vi "File Compatibility Test.vi"() -> (0 "error out":errorcluster, 3 "result":string)   [LabVIEW 2014]
doc: "This test will find some issues caused by a modification to To and From string methods that don't support older configuration versions. The test finds and attempts to open all .pcfg files that it can find in the repo and returns details in a 'result' string if any of them fail."
uses:
  <vilib>/NI/Configuration Framework/class discovery singleton/class discovery singleton methods.ctl
  <vilib>/NI/DCAF/Tag Editor Core/Configuration Editor/Classes/SystemConfigRepo/SystemConfigRepo.lvclass
  <vilib>/NI/DCAF/Tag Editor Core/Framework Configuration Classes/class cache/PL_class cache.lvlib
  <vilib>/NI/Configuration Framework/class discovery singleton/class discovery singleton.lvlib
panel:
  out "All Files in Dir":path[](array[path])
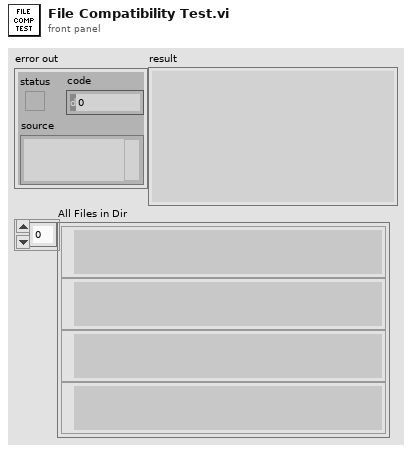
[diagram p1: front panel]
types:
  T1 = typedef "class discovery singleton.lvlib/class discovery singleton methods.ctl" = enum16{"add search paths", "load class by name", "list available classes", "get class path", "delete cache"}
  T2 = typedef "PL_class cache.lvlib/cache definition.ctl" = cluster{"configuration":T3, "class cache data":T4}
  T3 = typedef "PL_class cache.lvlib/cache search configuration.ctl" = cluster{"Search Paths":path[], "Folders to Exclude":string[], "full class list":path[]}
  T4 = typedef "PL_class cache.lvlib/cached class information.ctl" = cluster{"targets":T5[], "engines":T6[], "modules":T6[], "ignored class list":path[]}
  T5 = typedef "PL_class cache.lvlib/target class metadata.ctl" = cluster{"file name":string, "fully qualified name":string, "menu display name":string, "configuration class name":string}
  T6 = typedef "PL_class cache.lvlib/class metadata.ctl" = cluster{"file name":string, "fully qualified name":string, "menu display name":string, "configuration class":string, "category":string, "instances allowed":i32, "supported targets":T7[]}
  T7 = typedef "TBM configuration.lvclass/Target Types.ctl" = enum16{"Windows", "Mac", "Linux", "Linux RT ARM", "VxWorks", "Pharlap", "Other", "Linux RT x64"}
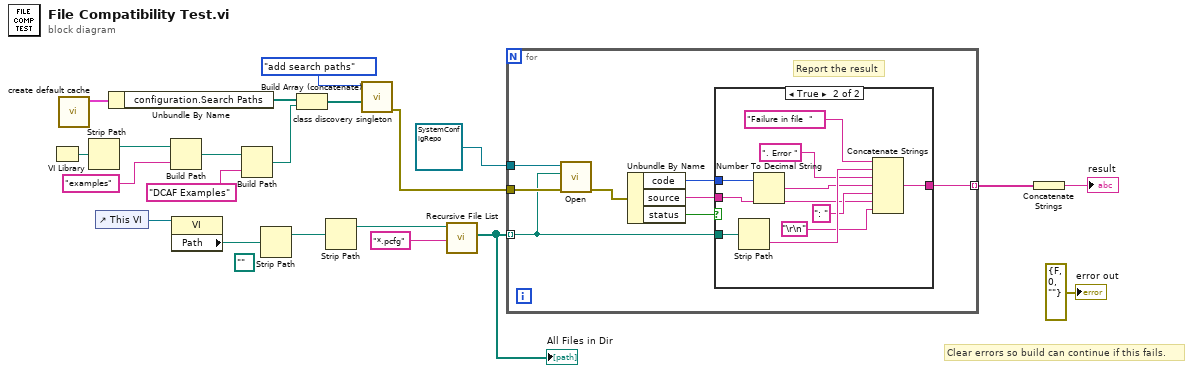
[diagram p0: block diagram]
diagram:
  (unwired) path "" ("VI Path")
  # "Clear errors so build can continue if this fails."
  n1 = VI Library() -> (path=w9:path)
  n2 = call <vilib>:"create default cache.vi"() -> ("cache"=w21:T2)  [unwired: 11 in]
  n3 = Strip Path(path=w9) -> (stripped path=w8:path)  [unwired: 1 out]
  n4 = control-ref of="This VI"() -> (w20:refnum<vi>)
  n5 = Unbundle By Name(w21) -> ("configuration.Search Paths"=w10:path[])
  n6 = Build Path(base path=w8, name or relative path="examples") -> (appended path=w6:path)
  n7 = property class="VI"(reference=w20) -> ("Path"=w19:path)  [unwired: 1 in, 2 out]
  n8 = Build Path(base path=w6, name or relative path="DCAF Examples") -> (appended path=w1:path)
  n9 = Strip Path(path=w19) -> (stripped path=w18:path)  [unwired: 1 out]
  n10 = Build Array (concatenate)(w10, w1) -> (w2:path[])
  n11 = Strip Path(path=w18) -> (stripped path=w17:path)  [unwired: 1 out]
  n12 = call <vilib>:"class discovery singleton.vi"("Plugin Search Paths"=w2, "method"=class_discovery_singleton_methods."add search paths") -> ("error out"=w3:errorcluster)  [unwired: 6 in, 3 out]
  n13 = call <vilib>:"Recursive File List.vi"("pattern"="*.pcfg", "Folder Path"=w17) -> ("All Files in Dir"=w15:path[])  [unwired: 5 in, 4 out]
  "All Files in Dir" <- w15
  n14 = for {
    tunnel: w3 -> [w29]
    tunnel: refnum<class "SystemConfigRepo.lvclass"> refnum ("repository out") -> [w28]
    tunnel: [w23] -> w13 mode=indexing
    tunnel: w15 -> [w22] mode=indexing
    # "Report the result"
    n15 = call-dynamic "Open.vi"("error in"=w29, "file path"=w22, "repository in"=w28) -> ("error out"=w27:errorcluster)  [unwired: 6 in, 2 out]
    n16 = Unbundle By Name(w27) -> ("code"=w25:i32, "source"=w24:string, "status"=w26:bool)
    n17 = case shown="True" w26 {
      tunnel: [_ w37] -> w23
      tunnel: w25 -> [_ w39]
      tunnel: w24 -> [_ w31]
      tunnel: w22 -> [_ w36]
      frame False {
      }
      frame True {
        n18 = Strip Path(path=w36) -> (name=w35:string)  [unwired: 1 out]
        n19 = Number To Decimal String(number=w39) -> (decimal integer string=w33:string)  [unwired: 1 in]
        n20 = Concatenate Strings("Failure in file  " ("string"), w35, ". Error " ("string"), w33, ": " ("string"), w31, "\r\n") -> (w37:string)
      }
    }
  }
  n21 = Concatenate Strings(w13) -> (→"result":string)
  "error out" <- errorcluster {"status"=FALSE, "code"=0, "source"=""} ("error out")
